vi "Farbanpassung.vi"(8 "error in (no error)":errorcluster caption="Fehler (Eingang, kein Fehler)", 10 "modal?":bool, 11 "Device ID":T2(ring)) -> (0 "error out":errorcluster caption="Fehler (Ausgang)", 2 "Farbwerte":T1={"Rot-min."=230.0, "Rot.max."=240.0, "Blau-min."=300.0, "Blau-max."=320.0, "Grün-min."=312.0, "Grün-max."=319.0, "Weiß-min."=220.0, "Weiß-max."=230.0}, 3 "Device ID Out":T2(ring))   [LabVIEW 2010]
uses:
  <vilib>/Utility/file.llb/Read From Spreadsheet File (DBL).vi
  <vilib>/Utility/file.llb/Write To Spreadsheet File (DBL).vi
panel:
  out "ende?":bool
  out "zwischen farbwerte":T1={"Rot-min."=1.0, "Rot.max."=12.0, "Blau-min."=2.0, "Blau-max."=22.0, "Grün-min."=3.0, "Grün-max."=32.0, "Weiß-min."=4.0, "Weiß-max."=42.0}
  out "Registerkarte":enum32{"Seite 1", "Seite 2", "Seite 3"}(tab)
  in  "test":bool
  in  "neue werte erstellen":bool
  in  "laden":bool
  in  "zurück":bool
  out "String 2":string
  in  "weiter":bool
  out "Aktueller Wert:":ext
  out "aktueeler wert schieberregler":ext(slide) scale=0.0..1032.0
  in  "speichern":bool
  out "bild-erkantte farbe":u16(ring) caption="Erkannte Farbe?"
  out "String 3":string
  in  "abbrechen":bool
  in  "ok":bool
  out "String":string
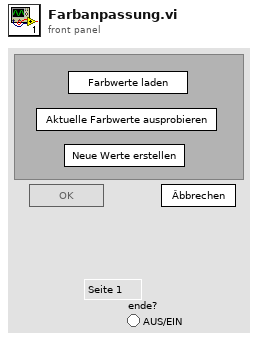
[diagram p1: front panel]
types:
  T1 = cluster{"Rot-min.":dbl, "Rot.max.":dbl, "Blau-min.":dbl, "Blau-max.":dbl, "Grün-min.":dbl, "Grün-max.":dbl, "Weiß-min.":dbl, "Weiß-max.":dbl}
  T2 = enum16{"Device 1", "Device 2", "Device 3", "Device 4", "Device 5", "Device 6", "Device 7", "Device 8"}
  T3 = enum8{"Input AX", "Input AY", "Input A1", "Input A2", "Input AZ", "Input AV", "Input D1", "Input D2", "Input AXR", "Input AYR"}
  T4 = enum8{"Robo Interface", "Extension 1", "Extension 2", "Extension 3"}
  T5 = enum8{"Input 1 (I1)", "Input 2 (I2)", "Input 3 (I3)", "Input 4 (I4)", "Input 5 (I5)", "Input 6 (I6)", "Input 7 (I7)", "Input 8 (I8)"}
  T6 = enum8{"Output 1 (O1)", "Output 2 (O2)", "Output 3 (O3)", "Output 4 (O4)", "Output 5 (O5)", "Output 6 (O6)", "Output 7 (O7)", "Output 8 (O8)"}
  T7 = enum16{"open", "replace", "create", "open or create", "replace or create", "replace or create with confirmation"}
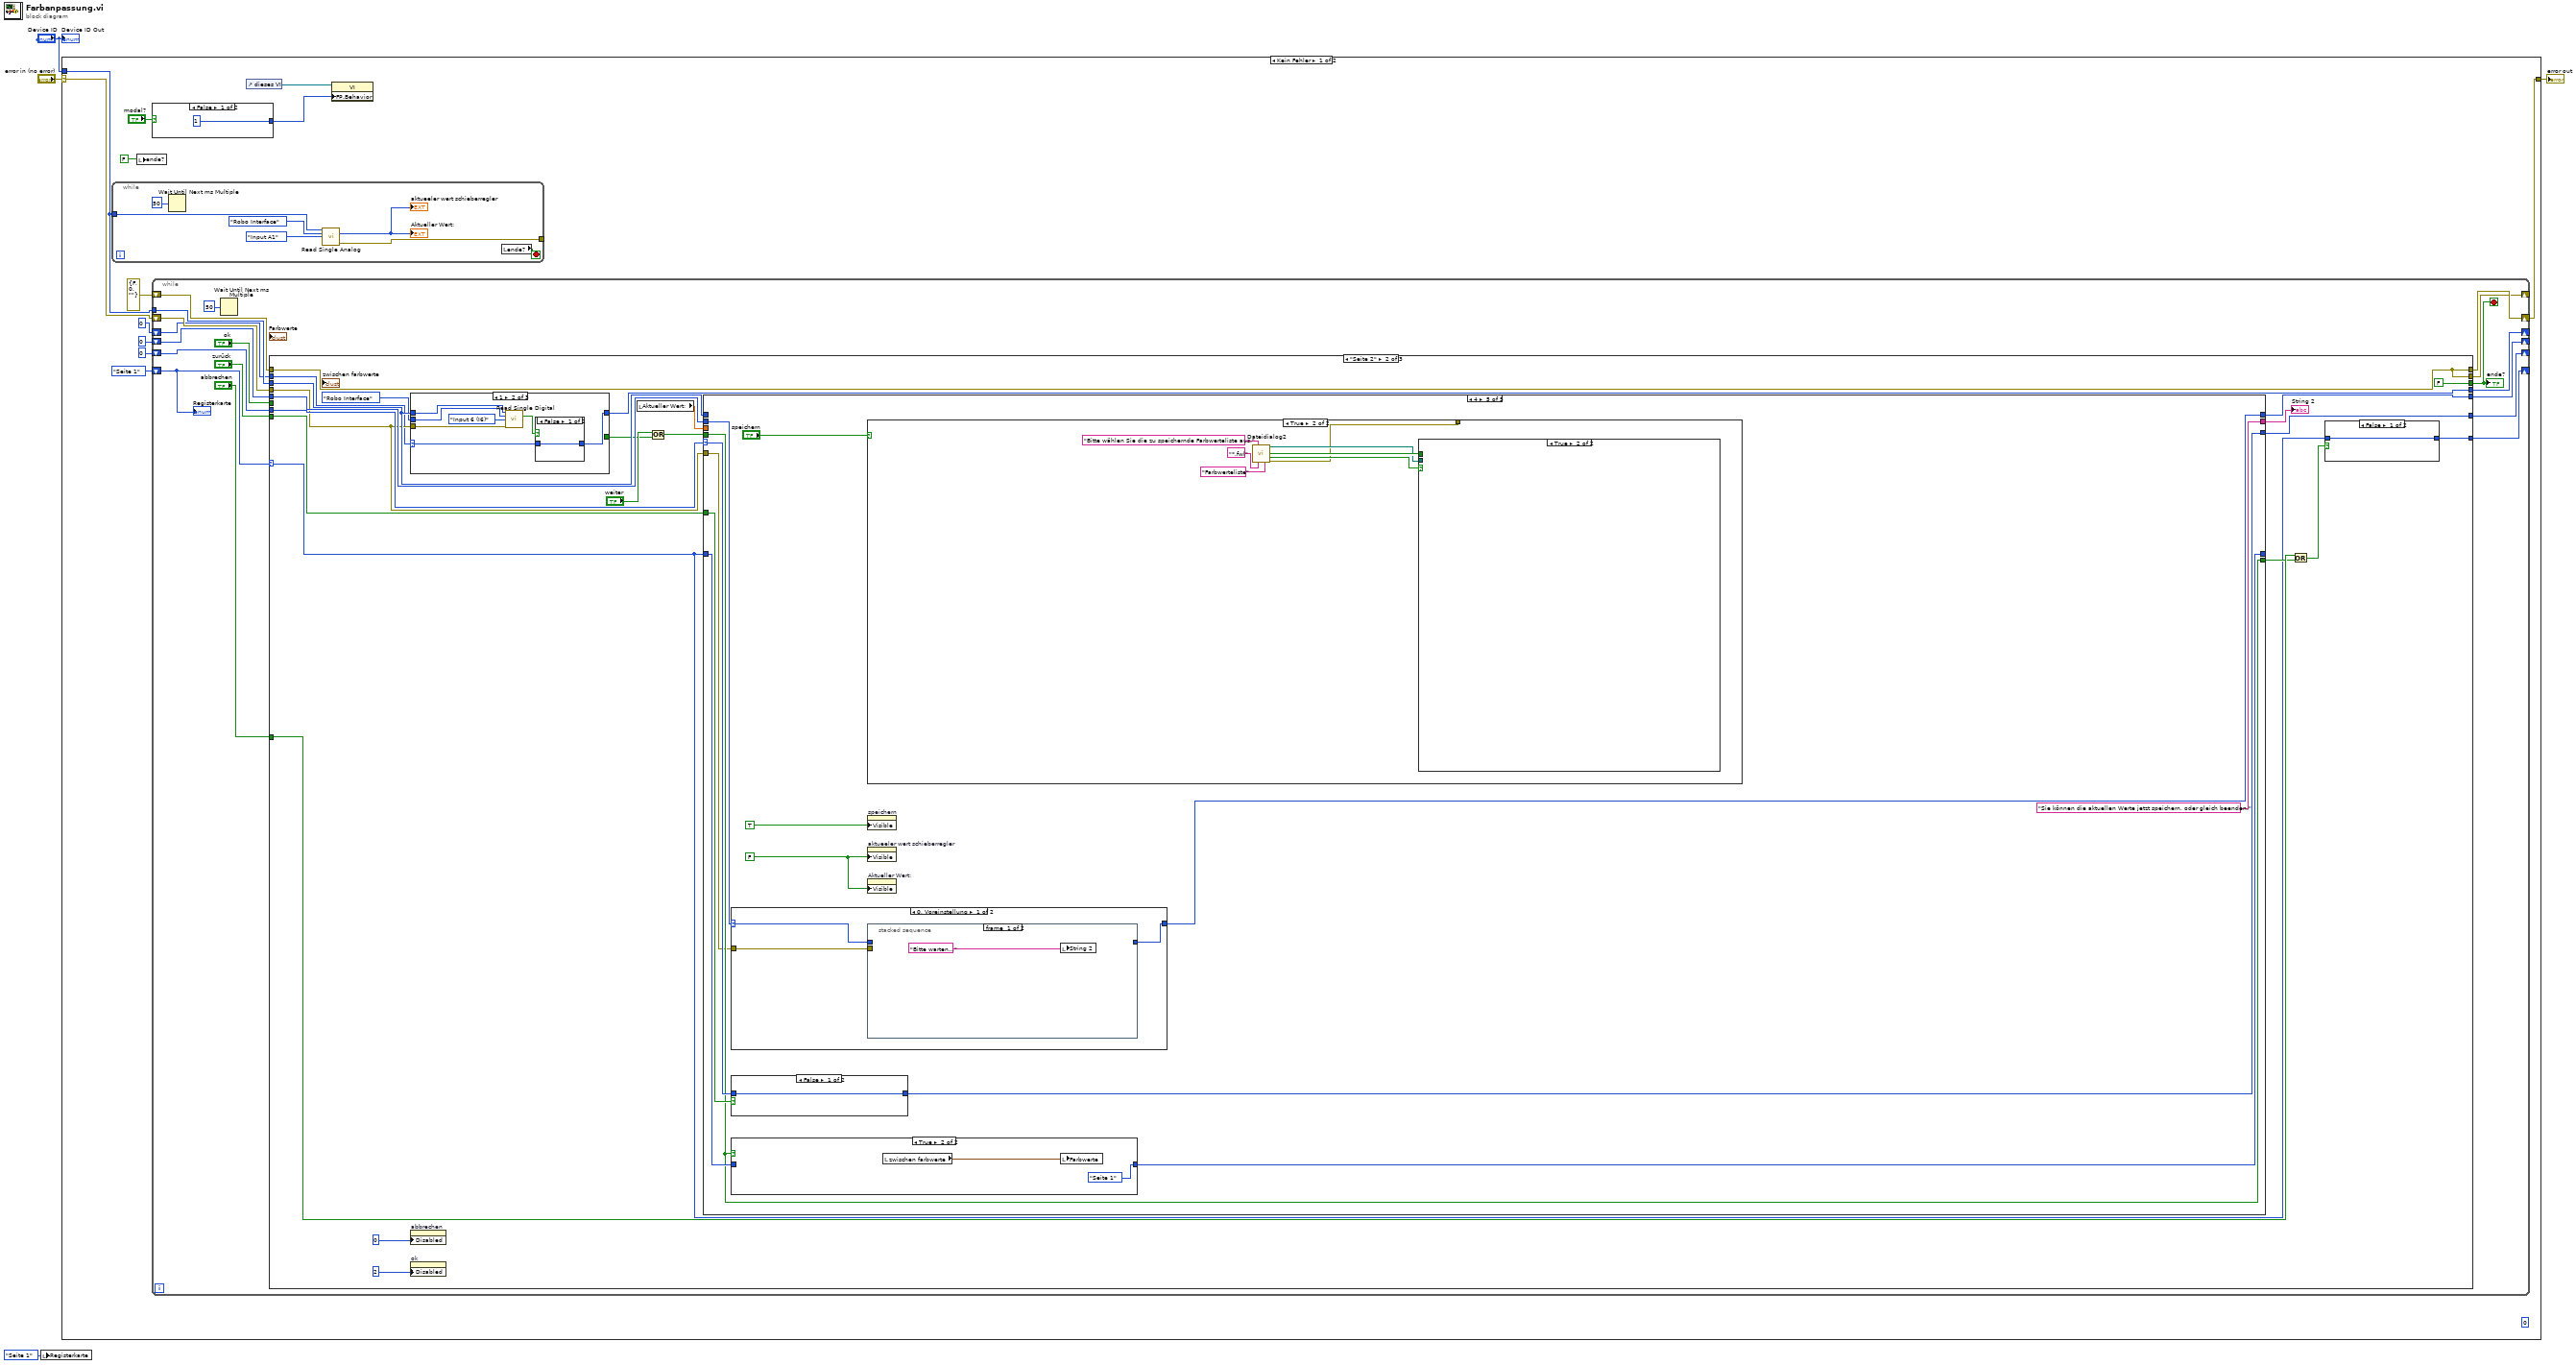
[diagram p0: block diagram]
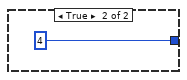
[diagram p2: hidden frame]
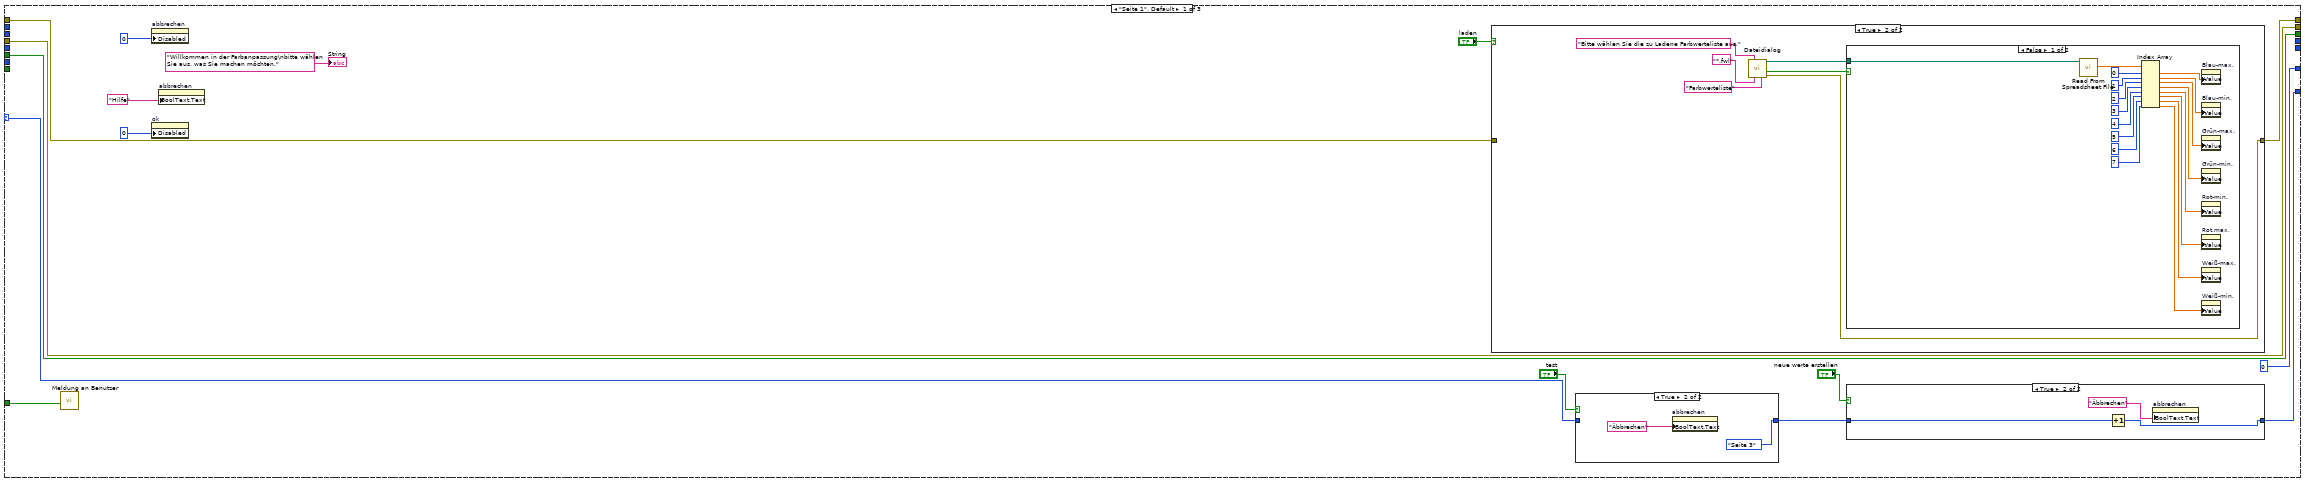
[diagram p3: hidden frame]
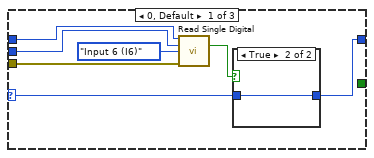
[diagram p8: hidden frame]
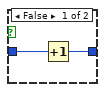
[diagram p9: hidden frame]
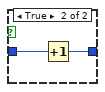
[diagram p10: hidden frame]
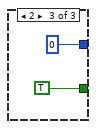
[diagram p11: hidden frame]
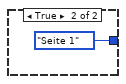
[diagram p12: hidden frame]
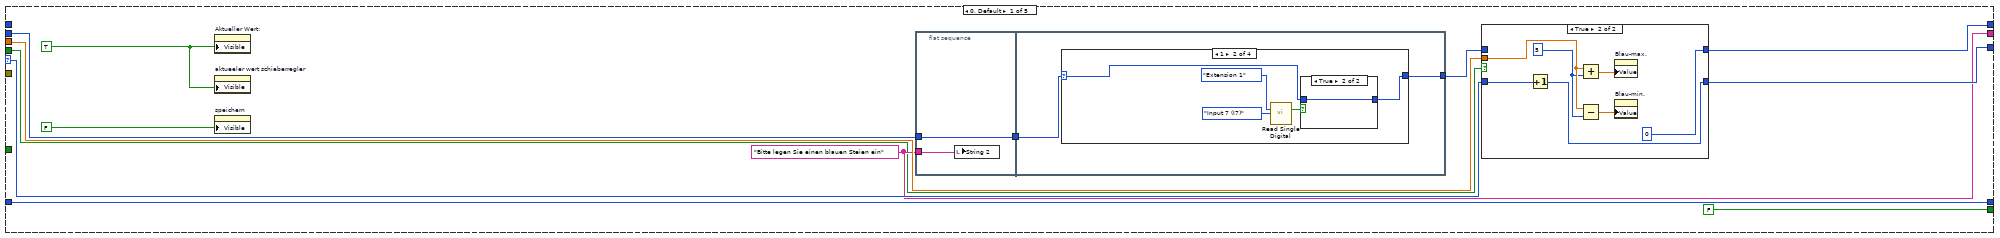
[diagram p13: hidden frame]
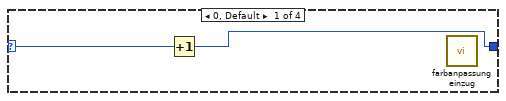
[diagram p14: hidden frame]
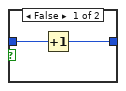
[diagram p15: hidden frame]
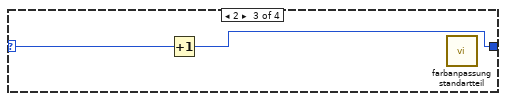
[diagram p16: hidden frame]
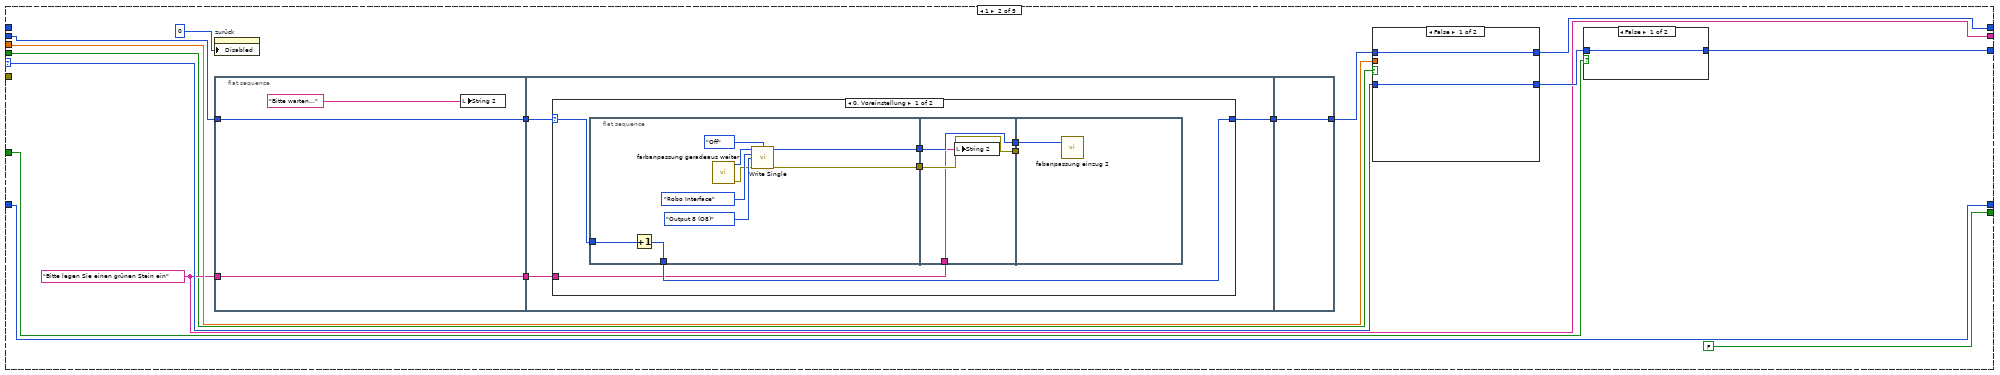
[diagram p19: hidden frame]
diagram:
  n1 = local write "Registerkarte"(enum32{"Seite 1", "Seite 2"}."Seite 1" ("Registerkarte")) -> ()
  n2 = case shown="Kein Fehler" "error in (no error)" {
    selector: "error in (no error)" -> [w16 w417]
    tunnel: "Device ID" -> [w5 _]
    tunnel: [w15 w417] -> w1
    frame No Error {
      (unwired) 0
      n3 = while {
        tunnel: [w18] -> _
        tunnel: w5 -> [w17]
        stop <- w23 stop-if-true
        n4 = Wait Until Next ms Multiple(millisecond multiple=50) -> ()  [unwired: 1 out]
        n5 = call "Read Single Analog.vi"("Device ID"=w17, "Module"=T4."Robo Interface", "Analog_Input"=T3."Input A1") -> ("Value"=→"aktueeler wert schieberregler" →"Aktueller Wert:":u16, "error out"=w18:errorcluster)  [unwired: 1 in, 10 out]
        n6 = local read "ende?"() -> (w23:bool)
      }
      n7 = local write "ende?"(FALSE) -> ()
      n8 = case shown="False" "modal?" {
        tunnel: [1 4] -> w8
        frame False {
        }
        frame True {
        }
      }
      n9 = while {
        tunnel: w5 -> [w42]
        shift-right: [w40] -> w15
        shift-left: w16 -> [w41]
        shift-right: [w39] -> _
        shift-left: enum32{"Seite 1", "Seite 2", "Seite 3"}."Seite 1" ("Registerkarte") -> [w33]
        shift-right: [w38] -> _
        shift-left: errorcluster {"status"=FALSE, "code"=0, "source"=""} ("error out") -> [w37]
        shift-right: [w35] -> _
        shift-left: 0 -> [w36]
        shift-right: [w28] -> _
        shift-left: 0 -> [w29]
        shift-right: [w27] -> _
        shift-left: 0 -> [w26]
        stop <- w34 stop-if-true
        n10 = Wait Until Next ms Multiple(millisecond multiple=50) -> ()  [unwired: 1 out]
        n11 = case shown="\"Seite 2\"" w33 {
          selector: w33 -> [w49 w102 w407]
          tunnel: w42 -> [_ w101 _]
          tunnel: w41 -> [w57 w99 w406]
          tunnel: [w57 w92 w406] -> w40
          tunnel: [w56 w107 w408] -> w39
          tunnel: [w54 w92 w405] -> w38
          tunnel: w37 -> [w53 w92 w405]
          tunnel: w36 -> [_ w115 w400]
          tunnel: [0 w114 w400] -> w35
          tunnel: [w51 FALSE ("ok") FALSE] -> w34
          tunnel: "ok" -> [w51 _ w399]
          tunnel: "zurück" -> [_ w96 _]
          tunnel: "abbrechen" -> [w44 w108 _]
          tunnel: w29 -> [_ w104 _]
          tunnel: [_ w103 _] -> w28
          tunnel: w26 -> [_ w95 _]
          tunnel: [_ w94 _] -> w27
          frame "Seite 1", Default {
            n12 = call "Meldung an Benutzer"("Enable"=w44) -> ()  [unwired: 2 in, 9 out]
            n13 = property on="abbrechen" class="Bool."("Disabled"=u8 0 ("Deaktiviert")) -> ()  [unwired: 2 in, 2 out]
            n14 = property on="ok" class="Bool."("Disabled"=u8 0 ("Deaktiviert")) -> ()  [unwired: 2 in, 2 out]
            n15 = property on="abbrechen" class="Bool."("BoolText.Text"="Hilfe" ("Boolescher Text.Text")) -> ()  [unwired: 2 in, 2 out]
            n16 = case shown="TRUE" "laden" {
              tunnel: [w67 w70] -> w54
              tunnel: w53 -> [w67 _]
              frame False {
              }
              frame True {
                n17 = call "Dateidialog"("prompt"="Bitte wählen Sie die zu Ladene Farbwerteliste aus.", "pattern (all files)"="*.fwl", "pattern label"="Farbwerteliste") -> ("selected path"=w68:path, "cancelled"=w69:bool, "error out"=w70:errorcluster)  [unwired: 4 in, 6 out]
                n18 = case shown="FALSE" w69 {
                  tunnel: w68 -> [w91 _]
                  frame False {
                    n19 = call-poly <vilib>:"Read From Spreadsheet File.vi"("file path (dialog if empty)"=w91) -> ("first row"=w82:dbl[])  [unwired: 3 in, 7 out]
                    n20 = Index Array(array=w82, index #1=0 ("Deaktivierter Index (Spalte)"), index #2=1 ("Deaktivierter Index (Spalte)"), index #3=2 ("Deaktivierter Index (Spalte)"), index #4=3 ("Deaktivierter Index (Spalte)"), index #5=4 ("Deaktivierter Index (Zeile)"), index #6=5 ("Deaktivierter Index (Zeile)"), index #7=6 ("Deaktivierter Index (Zeile)"), index #8=7 ("Deaktivierter Index (Zeile)")) -> (element #1=w90:dbl, element #2=w89:dbl, element #3=w88:dbl, element #4=w87:dbl, element #5=w86:dbl, element #6=w85:dbl, element #7=w84:dbl, element #8=w83:dbl)
                    n21 = property on="Blau-max." class="DigWert (strikt)"("Value"=w90) -> ()  [unwired: 2 in, 2 out]
                    n22 = property on="Blau-min." class="DigWert (strikt)"("Value"=w89) -> ()  [unwired: 2 in, 2 out]
                    n23 = property on="Grün-max." class="DigWert (strikt)"("Value"=w88) -> ()  [unwired: 2 in, 2 out]
                    n24 = property on="Grün-min." class="DigWert (strikt)"("Value"=w87) -> ()  [unwired: 2 in, 2 out]
                    n25 = property on="Rot-min." class="DigWert (strikt)"("Value"=w86) -> ()  [unwired: 2 in, 2 out]
                    n26 = property on="Rot.max." class="DigWert (strikt)"("Value"=w85) -> ()  [unwired: 2 in, 2 out]
                    n27 = property on="Weiß-max." class="DigWert (strikt)"("Value"=w84) -> ()  [unwired: 2 in, 2 out]
                    n28 = property on="Weiß-min." class="DigWert (strikt)"("Value"=w83) -> ()  [unwired: 2 in, 2 out]
                  }
                  frame True {
                  }
                }
              }
            }
            n29 = case shown="TRUE" "test" {
              tunnel: [w60 enum32{"Seite 1", "Seite 2", "Seite 3"}."Seite 3" ("Registerkarte")] -> w48
              tunnel: w49 -> [w60 _]
              frame False {
              }
              frame True {
                n30 = property on="abbrechen" class="Bool."("BoolText.Text"="Âbbrechen" ("Boolescher Text.Text")) -> ()  [unwired: 2 in, 2 out]
              }
            }
            n31 = case shown="TRUE" "neue werte erstellen" {
              tunnel: w48 -> [w63 w66]
              tunnel: [w63 w65] -> w56
              frame False {
              }
              frame True {
                n32 = Increment(x=w66) -> (x+1=w65:enum32{"Seite 1", "Seite 2", "Seite 3"})
                n33 = property on="abbrechen" class="Bool."("BoolText.Text"="Âbbrechen" ("Boolescher Text.Text")) -> ()  [unwired: 2 in, 2 out]
              }
            }
            "String" <- "Willkommen in der Farbanpassung\nbitte wählen Sie aus, was Sie machen möchten." ("String")
          }
          frame "Seite 2" {
            n34 = case shown="1" w95 {
              selector: w95 -> [w118 w127 _]
              tunnel: w101 -> [w122 w132 _]
              tunnel: T4."Robo Interface" ("Module") -> [w121 w131 _]
              tunnel: w99 -> [w119 w129 _]
              tunnel: [_ _ TRUE] -> w97
              tunnel: [w117 w126 0] -> w94
              frame 0, Default {
                n35 = call "Read Single Digital.vi"("Device ID"=w122, "Module"=w121, "Digital_Input"=T5."Input 6 (I6)", "error in"=w119) -> ("Value"=w116:bool)  [unwired: 11 out]
                n36 = case shown="TRUE" w116 {
                  tunnel: w118 -> [w124 w125]
                  tunnel: [w123 w125] -> w117
                  frame False {
                    n37 = Increment(x=w124) -> (x+1=w123:i32)
                  }
                  frame True {
                  }
                }
              }
              frame 1 {
                n38 = call "Read Single Digital.vi"("Device ID"=w132, "Module"=w131, "Digital_Input"=T5."Input 6 (I6)", "error in"=w129) -> ("Value"=w128:bool)  [unwired: 11 out]
                n39 = case shown="False" w128 {
                  tunnel: w127 -> [w133 w135]
                  tunnel: [w133 w134] -> w126
                  frame False {
                  }
                  frame True {
                    n40 = Increment(x=w135) -> (x+1=w134:i32)
                  }
                }
              }
              frame 2 {
              }
            }
            n41 = property on="abbrechen" class="Bool."("Disabled"=u8 0 ("Deaktiviert")) -> ()  [unwired: 2 in, 2 out]
            n42 = property on="ok" class="Bool."("Disabled"=u8 2 ("Deaktiviert")) -> ()  [unwired: 2 in, 2 out]
            n43 = local read "Aktueller Wert:"() -> (w93:ext)
            n44 = Or(x="weiter", y=w97) -> (x .or. y?=w98:bool)
            n45 = case shown="4" w115 {
              selector: w115 -> [w152 w194 w248 w303 w350]
              tunnel: w101 -> [_ _ _ _ _]
              tunnel: w99 -> [_ _ _ _ w345]
              tunnel: w93 -> [w151 w193 w247 w302 _]
              tunnel: [w147 w189 w242 w298 w349] -> w114
              tunnel: [w141 w182 w236 w289 "Sie können die aktuellen Werte jetzt speichern, oder gleich beenden."] -> w113
              tunnel: w98 -> [w140 w179 w245 w300 w346]
              tunnel: [w150 w192 w246 w301 w354] -> _
              tunnel: w102 -> [w150 w192 w246 w301 w353]
              tunnel: w96 -> [_ w191 w244 w297 w348]
              tunnel: [FALSE FALSE FALSE FALSE w346] -> w105
              tunnel: w104 -> [w145 w186 w240 w293 w344]
              tunnel: [w143 w184 w238 w291 w343] -> w103
              frame 0, Default {
                w149 = TRUE ("Sichtbar")
                w141 = "Bitte legen Sie einen blauen Steien ein"
                n46 = property on="Aktueller Wert:" class="DigWert (strikt)"("Visible"=w149) -> ()  [unwired: 2 in, 2 out]
                n47 = property on="aktueeler wert schieberregler" class="Schieber (strikt)"("Visible"=w149) -> ()  [unwired: 2 in, 2 out]
                n48 = property on="speichern" class="Bool."("Visible"=FALSE ("Sichtbar")) -> ()  [unwired: 2 in, 2 out]
                n49 = flat-sequence {
                  tunnel: w145 -> [w154]
                  tunnel: [w154] -> w142
                  tunnel: w141 -> [w153]
                  tunnel: [w155] -> w144
                  tunnel: w142 -> [w156]
                  frame #0 {
                    n50 = local write "String 2"(w153) -> ()
                  }
                  frame #1 {
                    n51 = case shown="1" w156 {
                      selector: w156 -> [w157 w159 w168 w169]
                      tunnel: [w158 w160 w167 w169] -> w155
                      frame 0, Default {
                        n52 = Increment(x=w157) -> (x+1=w158:i32)
                        n53 = call "farbanpassung einzug.vi"() -> ()  [unwired: 2 in, 10 out]
                      }
                      frame 1 {
                        n54 = call "Read Single Digital.vi"("Module"=T4."Extension 1", "Digital_Input"=T5."Input 7 (I7)") -> ("Value"=w161:bool)  [unwired: 2 in, 11 out]
                        n55 = case shown="TRUE" w161 {
                          tunnel: [w165 w166] -> w160
                          tunnel: w159 -> [w164 w166]
                          frame False {
                            n56 = Increment(x=w164) -> (x+1=w165:i32)
                          }
                          frame True {
                          }
                        }
                      }
                      frame 2 {
                        n57 = Increment(x=w168) -> (x+1=w167:i32)
                        n58 = call "farbanpassung standartteil.vi"() -> ()  [unwired: 2 in, 9 out]
                      }
                      frame 3 {
                      }
                    }
                  }
                }
                n59 = case shown="TRUE" w140 {
                  tunnel: w152 -> [w171 w178]
                  tunnel: w151 -> [_ w175]
                  tunnel: [w171 w176] -> w147
                  tunnel: w144 -> [w170 _]
                  tunnel: [w170 0] -> w143
                  frame False {
                  }
                  frame True {
                    w174 = u16 5 ("y")
                    n60 = Increment(x=w178) -> (x+1=w176:i32)
                    n61 = Add(x=w175, y=w174) -> (x+y=w177:ext)
                    n62 = Subtract(x=w175, y=w174) -> (x-y=w173:ext)
                    n63 = property on="Blau-max." class="DigWert (strikt)"("Value"=w177) -> ()  [unwired: 2 in, 2 out]
                    n64 = property on="Blau-min." class="DigWert (strikt)"("Value"=w173) -> ()  [unwired: 2 in, 2 out]
                  }
                }
              }
              frame 1 {
                w182 = "Bitte legen Sie einen grünen Stein ein"
                n65 = property on="zurück" class="Bool."("Disabled"=u8 0 ("Deaktiviert")) -> ()  [unwired: 2 in, 2 out]
                n66 = flat-sequence {
                  tunnel: w186 -> [w197]
                  tunnel: [w197] -> w183
                  tunnel: w182 -> [w195]
                  tunnel: [w195] -> w180
                  tunnel: w183 -> [w200]
                  tunnel: [w199] -> w181
                  tunnel: w180 -> [w198]
                  tunnel: [w222] -> w185
                  tunnel: w181 -> [w222]
                  frame #0 {
                    n67 = local write "String 2"("Bitte warten..." ("String 2")) -> ()
                  }
                  frame #1 {
                    n68 = case shown="0, Voreinstellung" w200 {
                      selector: w200 -> [w207 w221]
                      tunnel: [w206 w221] -> w199
                      tunnel: w198 -> [w203 _]
                      frame 0, Default {
                        n69 = flat-sequence {
                          tunnel: w207 -> [w216]
                          tunnel: [w215] -> w206
                          tunnel: [w210] -> w205
                          tunnel: [w208] -> w204
                          tunnel: w205 -> [w219]
                          tunnel: w204 -> [w218]
                          tunnel: w203 -> [w217]
                          tunnel: [w219] -> w202
                          tunnel: [w218] -> w201
                          tunnel: w202 -> [_]
                          tunnel: w201 -> [w220]
                          frame #0 {
                            n70 = Increment(x=w216) -> (x+1=w215:i32)
                            n71 = call "farbanpassung geradeaus weiter.vi"() -> ("error out"=w211:errorcluster, "Device ID Out"=w209:T2)  [unwired: 2 in, 8 out]
                            n72 = call "Write Single.vi"("Device ID"=w209, "Output_Action"=enum8{"Off", "On"}."Off", "Module"=T4."Robo Interface", "Single_Output"=T6."Output 8 (O8)", "error in"=w211) -> ("Device ID Out"=w208:T2, "error out"=w210:errorcluster)  [unwired: 1 in, 8 out]
                          }
                          frame #1 {
                            n73 = local write "String 2"(w217) -> ()
                          }
                          frame #2 {
                            n74 = call "fabanpassung einzug 2.vi"("Device ID Out"=w220) -> ()  [unwired: 1 in, 1 out]
                          }
                        }
                      }
                      frame 1 {
                      }
                    }
                  }
                  frame #2 {
                  }
                }
                n75 = case shown="FALSE" w179 {
                  tunnel: w194 -> [w227 w234]
                  tunnel: w193 -> [_ w231]
                  tunnel: [w227 w232] -> w190
                  tunnel: w185 -> [w226 _]
                  tunnel: [w226 0] -> w184
                  frame False {
                  }
                  frame True {
                    w230 = u16 5 ("y")
                    n76 = Increment(x=w234) -> (x+1=w232:i32)
                    n77 = Add(x=w231, y=w230) -> (x+y=w233:ext)
                    n78 = Subtract(x=w231, y=w230) -> (x-y=w229:ext)
                    n79 = property on="Grün-max." class="DigWert (strikt)"("Value"=w233) -> ()  [unwired: 2 in, 2 out]
                    n80 = property on="Grün-min." class="DigWert (strikt)"("Value"=w229) -> ()  [unwired: 2 in, 2 out]
                  }
                }
                n81 = case shown="FALSE" w191 {
                  tunnel: w190 -> [w223 w225]
                  tunnel: [w223 w224] -> w189
                  frame False {
                  }
                  frame True {
                    n82 = Decrement(x=w225) -> (x-1=w224:i32)
                  }
                }
              }
              frame 2 {
                w236 = "Bitte legen Sie einen roten Stein ein"
                n83 = flat-sequence {
                  tunnel: w240 -> [w251]
                  tunnel: [w251] -> w237
                  tunnel: w236 -> [w249]
                  tunnel: [w249] -> w235
                  tunnel: [w253] -> w239
                  tunnel: w237 -> [w254]
                  tunnel: w235 -> [w252]
                  frame #0 {
                    n84 = local write "String 2"("Bitte warten...") -> ()
                  }
                  frame #1 {
                    n85 = case shown="0, Voreinstellung" w254 {
                      selector: w254 -> [w260 w275]
                      tunnel: [w261 w275] -> w253
                      tunnel: w252 -> [w256 _]
                      frame 0, Default {
                        n86 = flat-sequence {
                          tunnel: w260 -> [w262]
                          tunnel: [w270] -> w259
                          tunnel: [w264] -> w258
                          tunnel: [w263] -> w257
                          tunnel: [w272] -> w255
                          tunnel: [w273] -> _
                          tunnel: [w274] -> w261
                          tunnel: w259 -> [w274]
                          tunnel: w258 -> [w273]
                          tunnel: w257 -> [w272]
                          tunnel: w256 -> [w271]
                          frame #0 {
                            n87 = Increment(x=w262) -> (x+1=w270:i32)
                            n88 = call "farbanpassung geradeaus weiter.vi"() -> ("error out"=w265:errorcluster, "Device ID Out"=w266:T2)  [unwired: 2 in, 8 out]
                            n89 = call "Write Single.vi"("Device ID"=w266, "Output_Action"=enum8{"Off", "On"}."Off", "Module"=T4."Robo Interface", "Single_Output"=T6."Output 8 (O8)", "error in"=w265) -> ("Device ID Out"=w263:T2, "error out"=w264:errorcluster)  [unwired: 1 in, 8 out]
                          }
                          frame #1 {
                            n90 = local write "String 2"(w271) -> ()
                          }
                        }
                        n91 = call "fabanpassung einzug 2.vi"("Device ID Out"=w255) -> ()  [unwired: 2 out]
                      }
                      frame 1 {
                      }
                    }
                  }
                }
                n92 = case shown="TRUE" w245 {
                  tunnel: w248 -> [w280 w287]
                  tunnel: w247 -> [_ w284]
                  tunnel: [w280 w285] -> w243
                  tunnel: w239 -> [w279 _]
                  tunnel: [w279 0] -> w238
                  frame False {
                  }
                  frame True {
                    w283 = u16 5 ("y")
                    n93 = Increment(x=w287) -> (x+1=w285:i32)
                    n94 = Add(x=w284, y=w283) -> (x+y=w286:ext)
                    n95 = Subtract(x=w284, y=w283) -> (x-y=w282:ext)
                    n96 = property on="Rot.max." class="DigWert (strikt)"("Value"=w286) -> ()  [unwired: 2 in, 2 out]
                    n97 = property on="Rot-min." class="DigWert (strikt)"("Value"=w282) -> ()  [unwired: 2 in, 2 out]
                  }
                }
                n98 = case shown="FALSE" w244 {
                  tunnel: w243 -> [w276 w278]
                  tunnel: [w276 w277] -> w242
                  frame False {
                  }
                  frame True {
                    n99 = Decrement(x=w278) -> (x-1=w277:i32)
                  }
                }
              }
              frame 3 {
                w296 = TRUE ("Sichtbar")
                w289 = "Bitte legen Sie einen weißen Stein ein"
                n100 = property on="aktueeler wert schieberregler" class="Schieber (strikt)"("Visible"=w296) -> ()  [unwired: 2 in, 2 out]
                n101 = property on="Aktueller Wert:" class="DigWert (strikt)"("Visible"=w296) -> ()  [unwired: 2 in, 2 out]
                n102 = property on="speichern" class="Bool."("Visible"=FALSE ("Sichtbar")) -> ()  [unwired: 2 in, 2 out]
                n103 = flat-sequence {
                  tunnel: w293 -> [w306]
                  tunnel: [w306] -> w290
                  tunnel: w289 -> [w305]
                  tunnel: [w305] -> w288
                  tunnel: [w308] -> w292
                  tunnel: w290 -> [w309]
                  tunnel: w288 -> [w307]
                  frame #0 {
                    n104 = local write "String 2"("Bitte warten...") -> ()
                  }
                  frame #1 {
                    n105 = case shown="0, Voreinstellung" w309 {
                      selector: w309 -> [w316 w330]
                      tunnel: [w315 w330] -> w308
                      tunnel: w307 -> [w311 _]
                      frame 0, Default {
                        n106 = flat-sequence {
                          tunnel: w316 -> [w325]
                          tunnel: [w324] -> w314
                          tunnel: [w318] -> w313
                          tunnel: [w317] -> w312
                          tunnel: [w327] -> w310
                          tunnel: [w328] -> _
                          tunnel: [w329] -> w315
                          tunnel: w314 -> [w329]
                          tunnel: w313 -> [w328]
                          tunnel: w312 -> [w327]
                          tunnel: w311 -> [w326]
                          frame #0 {
                            n107 = Increment(x=w325) -> (x+1=w324:i32)
                            n108 = call "geradeaus weiter.vi"() -> ("error out"=w319:errorcluster, "Device ID Out"=w320:T2)  [unwired: 3 in, 7 out]
                            n109 = call "Write Single.vi"("Device ID"=w320, "Output_Action"=enum8{"Off", "On"}."Off", "Module"=T4."Robo Interface", "Single_Output"=T6."Output 8 (O8)", "error in"=w319) -> ("Device ID Out"=w317:T2, "error out"=w318:errorcluster)  [unwired: 1 in, 8 out]
                          }
                          frame #1 {
                            n110 = local write "String 2"(w326) -> ()
                          }
                        }
                        n111 = call "fabanpassung einzug 2.vi"("Device ID Out"=w310) -> ()  [unwired: 2 out]
                      }
                      frame 1 {
                      }
                    }
                  }
                }
                n112 = case shown="FALSE" w300 {
                  tunnel: w303 -> [w335 w342]
                  tunnel: w302 -> [_ w339]
                  tunnel: [w335 w340] -> w299
                  tunnel: w292 -> [w334 _]
                  tunnel: [w334 0] -> w291
                  frame False {
                  }
                  frame True {
                    w338 = u16 5 ("y")
                    n113 = Increment(x=w342) -> (x+1=w340:i32)
                    n114 = Add(x=w339, y=w338) -> (x+y=w341:ext)
                    n115 = Subtract(x=w339, y=w338) -> (x-y=w337:ext)
                    n116 = property on="Weiß-max." class="DigWert (strikt)"("Value"=w341) -> ()  [unwired: 2 in, 2 out]
                    n117 = property on="Weiß-min." class="DigWert (strikt)"("Value"=w337) -> ()  [unwired: 2 in, 2 out]
                  }
                }
                n118 = case shown="FALSE" w297 {
                  tunnel: w299 -> [w331 w333]
                  tunnel: [w331 w332] -> w298
                  frame False {
                  }
                  frame True {
                    n119 = Decrement(x=w333) -> (x-1=w332:i32)
                  }
                }
              }
              frame 4 {
                w352 = FALSE ("Sichtbar")
                n120 = case shown="0, Voreinstellung" w344 {
                  selector: w344 -> [w356 w369]
                  tunnel: w345 -> [w358 _]
                  tunnel: [w357 w369] -> w343
                  frame 0, Default {
                    n121 = stacked-sequence {
                      tunnel: w358 -> [_ w367]
                      tunnel: [_ w366] -> w357
                      tunnel: w356 -> [_ w365]
                      frame #0 {
                        n122 = local write "String 2"("Bitte warten..." ("String 2")) -> ()
                      }
                      frame #1 {
                        n123 = call "geradeaus weiter.vi"("error in (no error)"=w367, "fehlbearbeitung?"=FALSE) -> ("error out"=w364:errorcluster, "Device ID Out"=w363:T2)  [unwired: 1 in, 7 out]
                        n124 = Increment(x=w365) -> (x+1=w366:i32)
                        n125 = call "Write Single.vi"("Device ID"=w363, "Output_Action"=enum8{"Off", "On"}."Off", "Module"=T4."Robo Interface", "Single_Output"=T6."Output 8 (O8)", "error in"=w364) -> ()  [unwired: 1 in, 10 out]
                      }
                    }
                  }
                  frame 1 {
                  }
                }
                n126 = case shown="False" w348 {
                  tunnel: w350 -> [w370 w372]
                  tunnel: [w370 w371] -> w349
                  frame False {
                  }
                  frame True {
                    n127 = Decrement(x=w372) -> (x-1=w371:i32)
                  }
                }
                n128 = case shown="True" w346 {
                  tunnel: [w396 enum32{"Seite 1", "Seite 2"}."Seite 1" ("Registerkarte")] -> w354
                  tunnel: w353 -> [w396 _]
                  frame False {
                  }
                  frame True {
                    n129 = local read "zwischen farbwerte"() -> (w398:T1)
                    n130 = local write "Farbwerte"(w398) -> ()
                  }
                }
                n131 = case shown="True" "speichern" {
                  tunnel: [_ w373] -> _
                  frame False {
                  }
                  frame True {
                    n132 = call "Dateidialog2"("prompt"="Bitte wählen Sie die zu speichernde Farbwerteliste aus.", "pattern (all files)"="*.fwl", "pattern label"="Farbwerteliste") -> ("selected path"=w375:path, "exists"=w376:bool, "cancelled"=w377:bool, "error out"=w373:errorcluster)  [unwired: 4 in, 5 out]
                    n133 = case shown="True" w377 {
                      tunnel: w376 -> [w392 _]
                      tunnel: w375 -> [w391 _]
                      frame False {
                        n134 = case shown="False" w392 {
                          tunnel: w391 -> [w393 w395]
                          tunnel: [w393 w395] -> w390
                          frame False {
                            n135 = Open/Create/Replace File(file path (use dialog)=w393, operation (0:open)=T7."create" ("Operation (0:Öffnen)")) -> ()  [unwired: 1 in, 6 out]
                          }
                          frame True {
                          }
                        }
                        n136 = property on="Blau-max." class="DigWert (strikt)"() -> ("Value"=w389:dbl)  [unwired: 2 in, 2 out]
                        n137 = property on="Grün-min." class="DigWert (strikt)"() -> ("Value"=w386:dbl)  [unwired: 2 in, 2 out]
                        n138 = property on="Rot-min." class="DigWert (strikt)"() -> ("Value"=w385:dbl)  [unwired: 2 in, 2 out]
                        n139 = property on="Rot.max." class="DigWert (strikt)"() -> ("Value"=w384:dbl)  [unwired: 2 in, 2 out]
                        n140 = property on="Weiß-min." class="DigWert (strikt)"() -> ("Value"=w382:dbl)  [unwired: 2 in, 2 out]
                        n141 = property on="Blau-min." class="DigWert (strikt)"() -> ("Value"=w388:dbl)  [unwired: 2 in, 2 out]
                        n142 = property on="Grün-max." class="DigWert (strikt)"() -> ("Value"=w387:dbl)  [unwired: 2 in, 2 out]
                        n143 = property on="Weiß-max." class="DigWert (strikt)"() -> ("Value"=w383:dbl)  [unwired: 2 in, 2 out]
                        n144 = Build Array(w389, w388, w387, w386, w385, w384, w383, w382) -> (w381:dbl[])
                        n145 = call-poly <vilib>:"Write To Spreadsheet File.vi"("append to file? (new file:F)"=FALSE, "1D data"=w381, "file path (dialog if empty)"=w390) -> ()  [unwired: 3 in, 3 out]
                      }
                      frame True {
                      }
                    }
                  }
                }
                n146 = property on="speichern" class="Bool."("Visible"=TRUE ("Sichtbar")) -> ()  [unwired: 2 in, 2 out]
                n147 = property on="aktueeler wert schieberregler" class="Schieber (strikt)"("Visible"=w352) -> ()  [unwired: 2 in, 2 out]
                n148 = property on="Aktueller Wert:" class="DigWert (strikt)"("Visible"=w352) -> ()  [unwired: 2 in, 2 out]
              }
            }
            "String 2" <- w113
            n149 = Or(x=w108, y=w105) -> (x .or. y?=w106:bool)
            n150 = case shown="False" w106 {
              tunnel: w102 -> [w138 _]
              tunnel: [w138 enum32{"Seite 1", "Seite 2", "Seite 3"}."Seite 1" ("Registerkarte")] -> w107
              frame False {
              }
              frame True {
              }
            }
          }
          frame "Seite 3" {
            # "0=blau\n1=rot\n2=weiß\n3=grün\n4=?"
            n151 = local read "Farbwerte"() -> (w403:T1)
            n152 = call "Farberkennung.vi"("Farbwerte"=w403) -> ("Farbe"=w402:u16)  [unwired: 2 in, 8 out]
            n153 = case shown="4" w402 {
              tunnel: [u16 0 ("bild-erkantte farbe") 2 3 ("bild-erkantte farbe") 4 ("bild-erkantte farbe") 1 ("bild-erkantte farbe")] -> w401
              frame 0, Default {
              }
              frame 1 {
              }
              frame 2 {
              }
              frame 3 {
              }
              frame 4 {
              }
            }
            "bild-erkantte farbe" <- w401
            n154 = case shown="FALSE" w399 {
              tunnel: [w415 enum32{"Seite 1", "Seite 2", "Seite 3"}."Seite 1" ("Registerkarte")] -> w408
              tunnel: w407 -> [w415 _]
              frame False {
              }
              frame True {
              }
            }
            "String 3" <- "Bitte legen Sie einen Stein ein" ("String 3")
          }
        }
        "ende?" <- w34
        "Registerkarte" <- w33
      }
      n155 = control-ref of="dieses VI"() -> (w10:refnum<vi>)
      n156 = property class="VI"(reference=w10, "FP.Behavior"=w8) -> ()  [unwired: 1 in, 2 out]
    }
    frame Error {
    }
  }
  "error out" <- w1
  "Device ID Out" <- "Device ID"
